vi "String - Search for [[  ]](2).vi"(10 "String":string, 11 "Strip \\00 (Unicode)":bool) -> (0 "after substring":string, 1 "before substring":string, 2 "matched string":string, 3 "Found":bool)   [LabVIEW 2013]
panel:
  # "The Quick [[Brown.Fox]] Jumps Over"
  # "Brown.Fox"
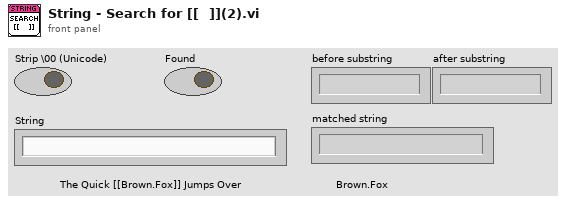
[diagram p1: front panel]
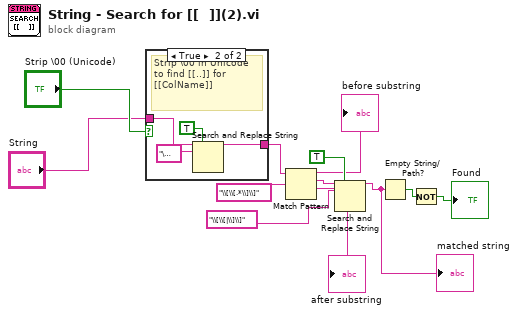
[diagram p0: block diagram]
diagram:
  n1 = case shown="True" "Strip \\00 (Unicode)" {
    tunnel: "String" -> [w13 w17]
    tunnel: [w13 w14] -> w8
    frame False {
    }
    frame True {
      # "Strip \\00 in Unicode\nto find [[..]] for [[ColName]]"
      n2 = Search and Replace String(replace all?=TRUE ("replace all? (F)"), input string=w17, search string="\u0000") -> (result string=w14:string)  [unwired: 5 in, 3 out]
    }
  }
  n3 = Match Pattern(string=w8, regular expression="\\[\\[.*\\]\\]") -> (before substring=→"before substring":string, match substring=w3:string, after substring=→"after substring":string)  [unwired: 1 in, 1 out]
  n4 = Search and Replace String(replace all?=TRUE ("replace all? (F)"), input string=w3, search string="\\[\\[|\\]\\]" ("substring (\"\")")) -> (result string=w7:string)  [unwired: 5 in, 3 out]
  "matched string" <- w7
  n5 = Empty String/Path?(string/path=w7) -> (empty?=w5:bool)
  n6 = Not(x=w5) -> (.not. x?=→"Found":bool)
